vi "SBG_Ellipse_skip_data_if_incorrect (SubVI) (1).vi"(2 "String":string, 4 "result string in":string) -> (1 "result string out":string)   [LabVIEW 2017]
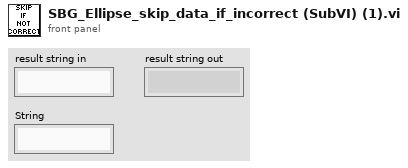
[diagram p1: front panel]
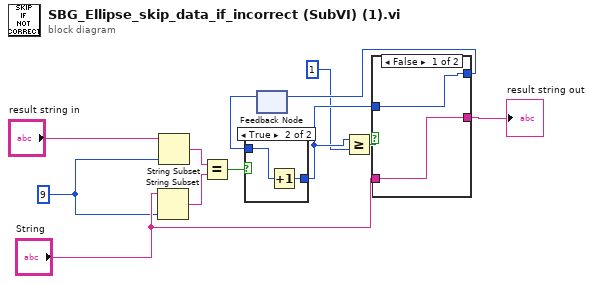
[diagram p0: block diagram]
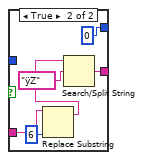
[diagram p2: hidden frame]
diagram:
  w3 = 9 ("length (rest)")
  n1 = String Subset(string="String", length (rest)=w3) -> (substring=w4:string)  [unwired: 1 in]
  n2 = String Subset(string="result string in", length (rest)=w3) -> (substring=w5:string)  [unwired: 1 in]
  n3 = Equal?(x=w5, y=w4) -> (x = y?=w6:bool)
  n4 = feedback #1() -> (w7:u32)  [unwired: 1 in]
  n5 = case shown="True" w6 {
    tunnel: [w13 w15] -> w10
    tunnel: w7 -> [w13 w14]
    frame False {
    }
    frame True {
      n6 = Increment(x=w14) -> (x+1=w15:u32)
    }
  }
  n7 = Greater Or Equal?(x=w10, y=u32 1) -> (x >= y?=w9:bool)
  n8 = case shown="False" w9 {
    tunnel: w10 -> [w16 _]
    tunnel: [w16 u32 0] -> w11
    tunnel: "String" -> [w17 w22]
    tunnel: [w17 w19] -> w1
    frame False {
    }
    frame True {
      n9 = Replace Substring(2:6 ("length (len. of substring)"), 5:w22) -> (1:w20:string)  [unwired: 2 in, 1 out]
      n10 = Search/Split String(string=w20, search string/char (-)="ÿZ") -> (match + rest of string=w19:string)  [unwired: 1 in, 2 out]
    }
  }
  "result string out" <- w1
  n11 = feedback-in #1(w11) -> ()
